vi "Update Item Value.vi"(7 "Section Name":string, 8 "error in (no error)":errorcluster, 9 "Value":string, 10 "Key Name":string, 11 "ODBC-Interface in":refnum<class "ODBC-Interface.lvclass">) -> (0 "error out":errorcluster, 2 "found":bool, 3 "ODBC-Interface out":refnum<class "ODBC-Interface.lvclass">)   [LabVIEW 2016, in "DB-Configuration.lvlib" / "ODBC-Interface.lvclass"]
doc: "Write boolean key value."
uses:
  ODBC-Interface.lvclass
  ODBC-Interface.lvclass/ODBC-Interface.ctl
  <vilib>/addons/database/Connection.llb/Conn Execute.vi
  <vilib>/addons/database/Recordset.llb/Rec Fetch Recordset Data (R).vi
  <vilib>/addons/database/Recordset.llb/Rec Destroy - Connection.vi
  <vilib>/addons/database/_DB Variant To Data/Database Variant To Data.xnode
  DB-Configuration.lvlib
  <vilib>/addons/database/NI_Database_API.lvlib
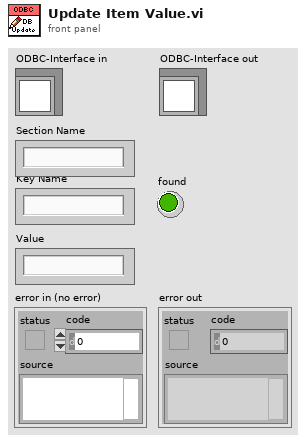
[diagram p1: front panel]
types:
  T1 = typedef "NI_Database_API.lvlib/Conn ObjectReference.ctl" = refnum<k1>
  T2 = typedef "NI_Database_API.lvlib/Rec ObjectReference.ctl" = refnum<k1>
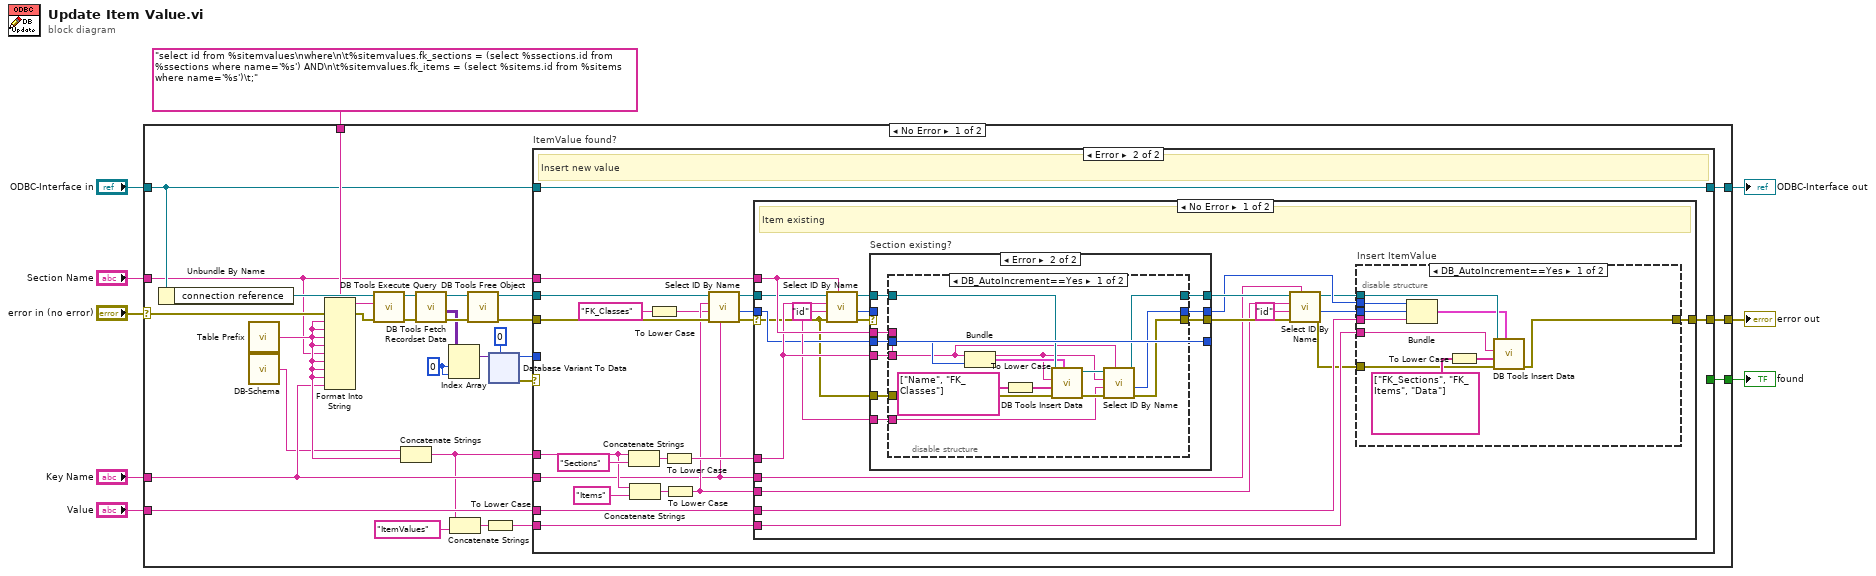
[diagram p0: block diagram]
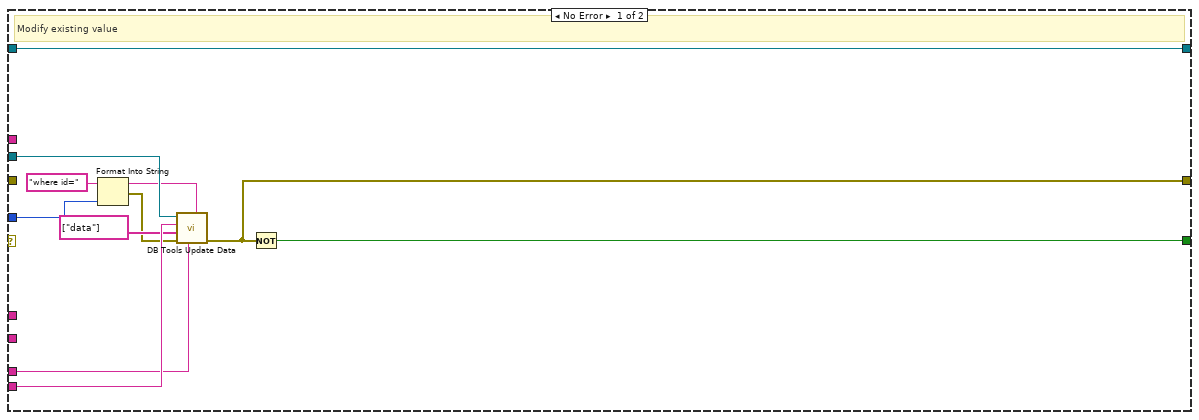
[diagram p2: hidden frame]
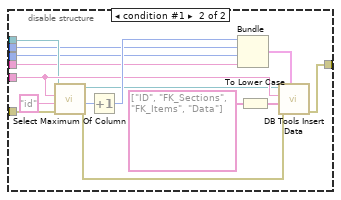
[diagram p3: hidden frame]
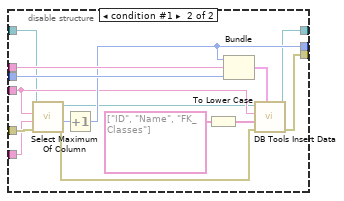
[diagram p5: hidden frame]
diagram:
  n1 = case shown="No Error" "error in (no error)" {
    selector: "error in (no error)" -> [w31 w192]
    tunnel: "ODBC-Interface in" -> [w17 w193]
    tunnel: "select id from %sitemvalues\nwhere\n\t%sitemvalues.fk_sections = (select %ssections.id from %ssections where name='%s') AND\n\t%sitemvalues.fk_items = (select %sitems.id from %sitems where name='%s')\t;" -> [w38 _]
    tunnel: [w26 w192] -> w3
    tunnel: [w18 w193] -> w8
    tunnel: "Section Name" -> [w15 _]
    tunnel: "Key Name" -> [w14 _]
    tunnel: [w19 _] -> w2
    tunnel: "Value" -> [w21 _]
    frame No Error {
      w30 = 0 ("index")
      n2 = Unbundle By Name(w17) -> ("connection reference"=w39:T1)
      n3 = call "Table Prefix.vi"() -> ("DB Table Prefix"=w16:string)
      n4 = call "DB-Schema.vi"() -> ("DB Schema (public.)"=w11:string)
      n5 = Format Into String(format string=w38, error in=w31, w16, w16, w16, w16, w15, w16, w16, w16, w14) -> (resulting string=w37:string, error out=w36:errorcluster)  [unwired: 1 in]
      n6 = call-poly <vilib>:"DB Tools Execute Query.vi"("error in (no error)"=w36, "SQL query"=w37, "connection reference"=w39) -> ("error out"=w34:errorcluster, "recordset reference"=w35:T2)  [unwired: 5 in]
      n7 = Concatenate Strings(w11, w16) -> (w10:string)
      n8 = call-poly <vilib>:"DB Tools Fetch Recordset Data.vi"("error in (no error)"=w34, "recordset reference"=w35) -> ("error out"=w33:errorcluster, "recordset data"=w29:variant[][], "recordset reference out"=w32:T2)  [unwired: 3 in]
      n9 = Index Array(array=w29, index (row)=w30, index (col)=w30) -> (element=w28:variant)
      n10 = Concatenate Strings(w10, "ItemValues" ("string")) -> (w24:string)
      n11 = call-poly <vilib>:"DB Tools Free Object.vi"("error in (no error)"=w33, "recordset reference"=w32) -> ("error out"=w12:errorcluster, "connection reference"=w27:T1)  [unwired: 8 in]
      n12 = To Lower Case(string=w24) -> (all lower case string=w23:string)
      n13 = xnode "Database Variant To Data"("database variant"=w28, "type"=0) -> ("data"=w20:i32, "error out"=w13:errorcluster)  [unwired: 1 in]
      n14 = case "ItemValue found?" shown="Error" w13 {
        tunnel: w27 -> [w50 w59]
        tunnel: [w41 w60] -> w26
        tunnel: w23 -> [w49 w62]
        tunnel: w21 -> [w47 w61]
        tunnel: w20 -> [w46 _]
        tunnel: [w40 _] -> w19
        tunnel: [w42 w65] -> w18
        tunnel: w17 -> [w42 w65]
        tunnel: w10 -> [_ w66]
        tunnel: w15 -> [_ w64]
        tunnel: w14 -> [_ w53]
        tunnel: w12 -> [_ w57]
        frame No Error {
          # "Modify existing value"
          n15 = Format Into String(initial string="where id=", w46) -> (resulting string=w44:string, error out=w43:errorcluster)  [unwired: 2 in]
          n16 = call <vilib>:"DB Tools Update Data.vi"("condition"=w44, "data"=w47, "error in (no error)"=w43, "columns"=string[] ["data"], "table"=w49, "connection reference"=w50) -> ("error out"=w41:errorcluster)  [unwired: 4 in, 1 out]
          n17 = Not(x=w41) -> (.not. x?=w40:bool)
        }
        frame Error {
          # "Insert new value"
          n18 = Concatenate Strings(w66, "Sections" ("string")) -> (w70:string)
          n19 = Concatenate Strings(w66, "Items" ("string")) -> (w68:string)
          n20 = To Lower Case(string="FK_Classes" ("Column (id)")) -> (all lower case string=w54:string)
          n21 = To Lower Case(string=w70) -> (all lower case string=w63:string)
          n22 = To Lower Case(string=w68) -> (all lower case string=w56:string)
          n23 = call "Select ID By Name.vi"("Name"=w53, "Error In"=w57, "Column (id)"=w54, "Table"=w56, "connection reference"=w59) -> ("Error Out"=w51:errorcluster, "ID"=w52:i32, "dup connection reference"=w58:T1)  [unwired: 4 in]
          n24 = case shown="No Error" w51 {
            selector: w51 -> [w71 w159]
            tunnel: w64 -> [w88 _]
            tunnel: w63 -> [w87 _]
            tunnel: w62 -> [w82 _]
            tunnel: w61 -> [w80 _]
            tunnel: [w79 w159] -> w60
            tunnel: w58 -> [w75 _]
            tunnel: w56 -> [w74 _]
            tunnel: w53 -> [w73 _]
            tunnel: w52 -> [w72 _]
            frame No Error {
              w83 = "id" ("Column (id)")
              # "Item existing"
              n25 = call "Select ID By Name.vi"("Name"=w88, "Error In"=w71, "Column (id)"=w83, "Table"=w87, "connection reference"=w75) -> ("Error Out"=w91:errorcluster, "ID"=w89:i32, "dup connection reference"=w90:T1)  [unwired: 4 in]
              n26 = case "Section existing?" shown="Error" w91 {
                selector: w91 -> [w117 _]
                tunnel: w89 -> [w120 _]
                tunnel: w90 -> [w119 w129]
                tunnel: [w120 w127] -> w81
                tunnel: w87 -> [_ w128]
                tunnel: w71 -> [_ w126]
                tunnel: w72 -> [w118 w124]
                tunnel: w88 -> [_ w125]
                tunnel: [w119 w123] -> w86
                tunnel: [w118 w124] -> _
                tunnel: [w117 w122] -> w85
                tunnel: w83 -> [_ w121]
                frame No Error {
                }
                frame Error {
                  n27 = disable-structure shown="DB_AutoIncrement==Yes" {
                    disable-tunnel: w129 -> [w143 w149]
                    disable-tunnel: w128 -> [w133 w151]
                    disable-tunnel: w126 -> [w140 w147]
                    disable-tunnel: w125 -> [w132 w156]
                    disable-tunnel: w124 -> [w139 w155]
                    disable-tunnel: [w137 w153] -> w127
                    disable-tunnel: [w135 w152] -> w122
                    disable-tunnel: [w131 w145] -> w123
                    disable-tunnel: w121 -> [w130 w144]
                    frame condition #0 (active) {
                      n28 = Bundle("Section Name"=w132, "ID"=w139) -> (w138:cluster{"Section Name":string, "ID":i32})  [unwired: 1 in]
                      n29 = To Lower Case(string=string[] ["Name", "FK_Classes"] ("columns")) -> (all lower case string=w141:string[])
                      n30 = call <vilib>:"DB Tools Insert Data.vi"("data"=w138, "error in (no error)"=w140, "columns"=w141, "table"=w133, "connection reference"=w143) -> ("error out"=w136:errorcluster, "connection reference out"=w134:T1)  [unwired: 5 in]
                      n31 = call "Select ID By Name.vi"("Name"=w132, "Error In"=w136, "Column (id)"=w130, "Table"=w133, "connection reference"=w134) -> ("Error Out"=w135:errorcluster, "ID"=w137:i32, "dup connection reference"=w131:T1)  [unwired: 4 in]
                    }
                    frame condition #1 {
                      n32 = call "Select Maximum Of Column.vi"("Error In"=w147, "Column Name (id)"=w144, "Table Name"=w151, "connection reference"=w149) -> ("Error Out"=w146:errorcluster, "Maximum"=w150:i32, "dup connection reference"=w148:T1)  [unwired: 5 in]
                      n33 = Increment(x=w150) -> (x+1=w153:i32)
                      n34 = To Lower Case(string=string[] ["ID", "Name", "FK_Classes"] ("columns")) -> (all lower case string=w157:string[])
                      n35 = Bundle(w153, "Section Name"=w156, "ID"=w155) -> (w154:cluster{i32, "Section Name":string, "ID":i32})  [unwired: 1 in]
                      n36 = call <vilib>:"DB Tools Insert Data.vi"("data"=w154, "error in (no error)"=w146, "columns"=w157, "table"=w151, "connection reference"=w148) -> ("error out"=w152:errorcluster, "connection reference out"=w145:T1)  [unwired: 5 in]
                    }
                  }
                }
              }
              n37 = call "Select ID By Name.vi"("Name"=w73, "Error In"=w85, "Column (id)"="id", "Table"=w74, "connection reference"=w86) -> ("Error Out"=w77:errorcluster, "ID"=w76:i32, "dup connection reference"=w78:T1)  [unwired: 4 in]
              n38 = disable-structure "Insert ItemValue" shown="DB_AutoIncrement==Yes" {
                disable-tunnel: w78 -> [w101 w110]
                disable-tunnel: w82 -> [w96 w112]
                disable-tunnel: w77 -> [w98 w108]
                disable-tunnel: w76 -> [w95 w102]
                disable-tunnel: [w92 w113] -> w79
                disable-tunnel: w81 -> [w94 w103]
                disable-tunnel: w80 -> [w93 w105]
                frame condition #0 (active) {
                  n39 = Bundle("ID"=w94, "ID"=w95, "Value"=w93) -> (w97:cluster{"ID":i32, "ID":i32, "Value":string})  [unwired: 1 in]
                  n40 = To Lower Case(string=string[] ["FK_Sections", "FK_Items", "Data"] ("columns")) -> (all lower case string=w99:string[])
                  n41 = call <vilib>:"DB Tools Insert Data.vi"("data"=w97, "error in (no error)"=w98, "columns"=w99, "table"=w96, "connection reference"=w101) -> ("error out"=w92:errorcluster)  [unwired: 5 in, 1 out]
                }
                frame condition #1 {
                  n42 = call "Select Maximum Of Column.vi"("Error In"=w108, "Column Name (id)"="id" ("Column (id)"), "Table Name"=w112, "connection reference"=w110) -> ("Error Out"=w107:errorcluster, "Maximum"=w111:i32, "dup connection reference"=w109:T1)  [unwired: 5 in]
                  n43 = Increment(x=w111) -> (x+1=w114:i32)
                  n44 = Bundle(w114, "ID"=w103, "ID"=w102, "Value"=w105) -> (w115:cluster{i32, "ID":i32, "ID":i32, "Value":string})  [unwired: 1 in]
                  n45 = To Lower Case(string=string[] ["ID", "FK_Sections", "FK_Items", "Data"] ("columns")) -> (all lower case string=w116:string[])
                  n46 = call <vilib>:"DB Tools Insert Data.vi"("data"=w115, "error in (no error)"=w107, "columns"=w116, "table"=w112, "connection reference"=w109) -> ("error out"=w113:errorcluster)  [unwired: 5 in, 1 out]
                }
              }
            }
            frame Error {
            }
          }
        }
      }
    }
    frame Error {
    }
  }
  "error out" <- w3
  "ODBC-Interface out" <- w8
  "found" <- w2
